vi "add module to engine.vi"(8 "error in":errorcluster, 10 "module ID":string, 11 "Standard Engine Configuration in":refnum<class "Standard Engine Configuration.lvclass">) -> (0 "error out":errorcluster, 3 "Standard Engine Configuration out":refnum<class "Standard Engine Configuration.lvclass">)   [LabVIEW 2013, in "Standard Engine Configuration.lvclass"]
uses:
  Standard Engine Configuration.lvclass
  Module Decimation.ctl
  Error Actions By Category.ctl
  <vilib>/NI/Tag Bus Module Framework/runtime/error classification.ctl
  Error Actions.ctl
  <vilib>/NI/Module Execution Interface/Engine Configuration/engine configuration.lvclass
  Standard Engine Configuration.lvclass/Standard Engine Configuration.ctl
  Module Specific Configuration.ctl
  Module Error Configuration.ctl
  <vilib>/NI/Tag Bus Module Framework/runtime/TBM module execution interface.lvclass
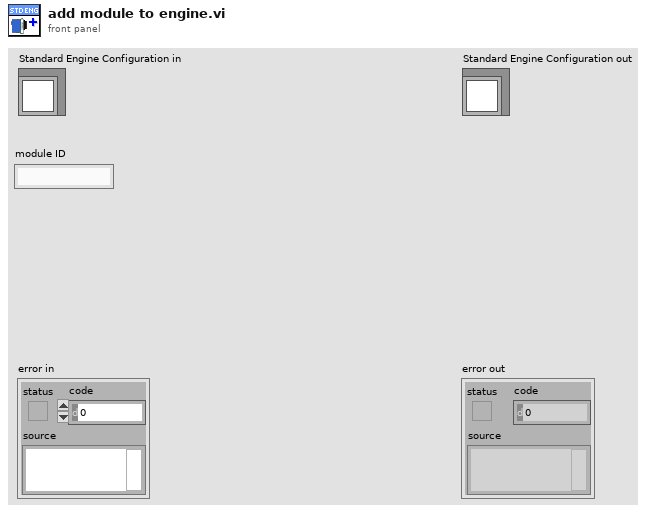
[diagram p1: front panel]
types:
  T1 = typedef "Standard Engine Configuration.lvclass/Error Actions By Category.ctl" = cluster{"error classification":T2, "Error Actions":T3[]}
  T2 = typedef "TBM module execution interface.lvclass/error classification.ctl" = enum16{"unknown", "none", "trivial", "recoverable", "critical"}
  T3 = typedef "Standard Engine Configuration.lvclass/Error Actions.ctl" = enum16{"Clear", "Notify", "Stop Component", "Stop Engine", "Safe State", "Attempt Recovery"}
  T4 = typedef "Standard Engine Configuration.lvclass/Module Decimation.ctl" = cluster{"Decimation":u16, "Offset":u16}
  T5 = typedef "Standard Engine Configuration.lvclass/Module Specific Configuration.ctl" = cluster{"Module ID":string, "Module Decimation":T4, "Module Error Configuration":T6, "execution order priority":i32}
  T6 = typedef "Standard Engine Configuration.lvclass/Module Error Configuration.ctl" = cluster{"Module Error Configuration":T1[]}
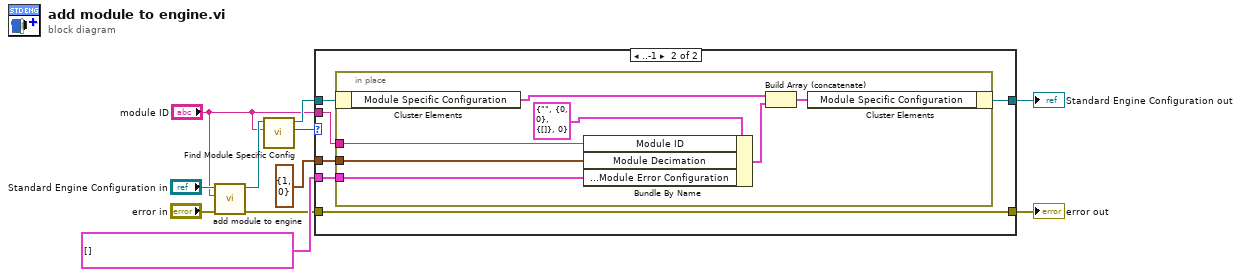
[diagram p0: block diagram]
diagram:
  n1 = call-parent "add module to engine.vi"("error in"="error in", "module ID"="module ID", "engine configuration in"="Standard Engine Configuration in") -> ("error out"=w4:errorcluster, "engine configuration out"=w2:refnum<class "Standard Engine Configuration.lvclass">)  [unwired: 7 in]
  n2 = call "Find Module Specific Config.vi"("Module ID"="module ID", "Standard Engine Repo Data in"=w2) -> ("Index"=w8:i32, "Standard Engine Repo Data out"=w10:refnum<class "Standard Engine Configuration.lvclass">)  [unwired: 8 in]
  n3 = case shown="..-1" w8 {
    tunnel: [w13 w19] -> w11
    tunnel: w10 -> [w13 w18]
    tunnel: w4 -> [w12 w17]
    tunnel: T4 {"Decimation"=1, "Offset"=0} ("module decimation") -> [_ w16]
    tunnel: T1[] [] ("Module Error Configuration") -> [_ w15]
    tunnel: [w12 w17] -> w5
    tunnel: "module ID" -> [_ w14]
    frame 0.. {
    }
    frame ..-1 {
      n4 = in-place {
        in-place-border: w16 -> [w22]
        in-place-border: w15 -> [w21]
        in-place-border: w14 -> [w20]
        n5 = in-place-cluster #1(w18) -> ("Module Specific Configuration"=w25:T5[])
        n6 = Bundle By Name(cluster=T5 {"Module ID"="", "Module Decimation"={"Decimation"=0, "Offset"=0}, "Module Error Configuration"={"Module Error Configuration"=[]}, "execution order priority"=0} ("Module Specific Configuration"), "Module ID"=w20, "Module Decimation"=w22, "Module Error Configuration.Module Error Configuration"=w21) -> (w23:T5)
        n7 = Build Array (concatenate)(w25, w23) -> (w24:T5[])
        n8 = in-place-cluster #1("Module Specific Configuration"=w24) -> (w19:refnum<class "Standard Engine Configuration.lvclass">)
      }
    }
  }
  "error out" <- w5
  "Standard Engine Configuration out" <- w11
